vi "PV-URL 2 PVConnectionObj.vi"(8 "Error In":errorcluster, 11 "PV":refnum<class "PV.lvclass">) -> (0 "Error Out":errorcluster, 2 "Success":bool, 3 "PVConnection":refnum<class "PVConnection.lvclass">)   [LabVIEW 2014, in "CS++ProcessVariables.lvlib"]
doc: "Return PV Connection object corresponding to PV protocol prefix."
uses:
  CS++ProcessVariables.lvlib
  ProcessVariable/PV.lvclass
  PVConnection/PVConnection.lvclass
  ProcessVariable/PV.lvclass/PV.ctl
  PVConnection/PVConnection.lvclass/PVConnection.ctl
  Libraries/Base/CS++Base.lvlib
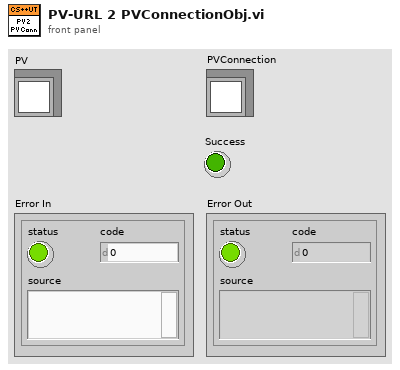
[diagram p1: front panel]
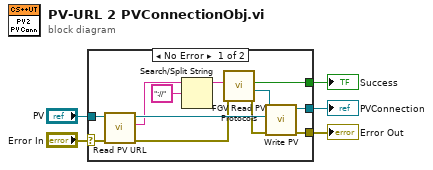
[diagram p0: block diagram]
diagram:
  n1 = case shown="No Error" "Error In" {
    selector: "Error In" -> [w9 w18]
    tunnel: [w13 _] -> w5
    tunnel: [w15 _] -> w4
    tunnel: [w6 w18] -> w3
    tunnel: "PV" -> [w10 _]
    frame No Error {
      n2 = call "Read PV URL.vi"("error in (no error)"=w9, "PV in"=w10) -> ("error out"=w8:errorcluster, "PV URL"=w11:string, "PV out"=w12:refnum<class "PV.lvclass">)  [unwired: 7 in]
      n3 = Search/Split String(string=w11, search string/char (-)="://") -> (substring before match=w16:string)  [unwired: 1 in, 2 out]
      n4 = call "FGV Read PV Protocols.vi"("Error In"=w8, "PV Protocol"=w16) -> ("Error Out"=w7:errorcluster, "PVConnection out"=w14:refnum<class "PVConnection.lvclass">, "Success"=w15:bool)  [unwired: 5 in, 2 out]
      n5 = call "Write PV.vi"("error in (no error)"=w7, "PV"=w12, "PVConnection in"=w14) -> ("error out"=w6:errorcluster, "PVConnection out"=w13:refnum<class "PVConnection.lvclass">)  [unwired: 7 in]
    }
    frame Error {
    }
  }
  "PVConnection" <- w5
  "Error Out" <- w3
  "Success" <- w4
